vi "Serve Control Endpoint.vi"(5 "Response":refnum<class "Response.lvclass">, 7 "Request":refnum<class "Request.lvclass">, 8 "error in (no error)":errorcluster) -> (0 "error out":errorcluster, 2 "Handled?":bool)   [LabVIEW 2023, in "Server.lvclass"]
uses:
  Server.lvclass
  Request/Request.lvclass
  Response/Response.lvclass
  Response/Standard Response Messages.ctl
  e9d03b97-7d0a-453d-8c8e-3f8556095b4f.vi
  1685da64-af02-4367-9c77-a6898df52c71.vi
  d533b881-5725-4b61-bb0f-1b9536aa055f.vi
  68d5b38b-bcce-484c-a16b-74d95231e072.vi
  96f92e60-dc3c-449d-a1e9-fb4d73dbd9f4.vi
  e9d03b97-7d0a-453d-8c8e-3f8556095b4f.vi/bf0030c7-b76b-4182-9f9e-16cd2e366061.vi
  1685da64-af02-4367-9c77-a6898df52c71.vi/bf0030c7-b76b-4182-9f9e-16cd2e366061.vi
  d533b881-5725-4b61-bb0f-1b9536aa055f.vi/bf0030c7-b76b-4182-9f9e-16cd2e366061.vi
  68d5b38b-bcce-484c-a16b-74d95231e072.vi/bf0030c7-b76b-4182-9f9e-16cd2e366061.vi
  96f92e60-dc3c-449d-a1e9-fb4d73dbd9f4.vi/bf0030c7-b76b-4182-9f9e-16cd2e366061.vi
  Request/Get Request.vi
  Response/Set Body.vi
  Response/Set Content Type.vi
  Response/Set Status Code.vi
  Response/Send.vi
  Response/Private/Format Control Data Element.vi
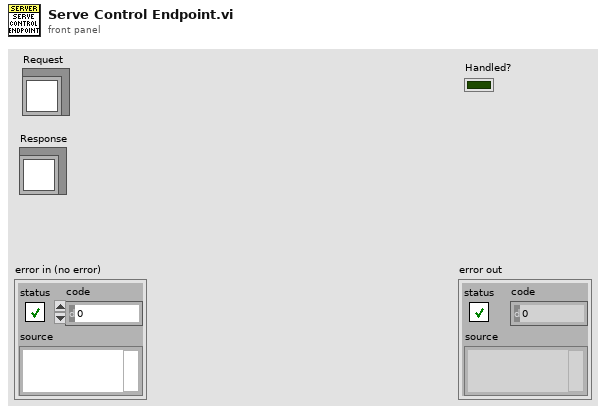
[diagram p1: front panel]
types:
  T1 = typedef "Server.lvclass/ObjectAttributes.ctl" = cluster{"Static Data":path, "MIME Types":variant, "Shutdown":bool, "API Queue":refnum<queue>, "ControlEndpoints":map{string, cluster{"Ref":refnum<vi>, "Mode":T2}}, "EventEndpoints":map{string, refnum<user-event>}}
  T2 = typedef "Server.lvclass/Control Ref Endpoint Access Mode.ctl" = enum16{"None", "Read/Write", "Read Only", "Write Only"}
  T3 = typedef "Request.ctl" = cluster{"Method":string, "URI":string, "Protocol":string, "Raw Path":string, "Query":string, "Fragment":string, "Raw Body":string, "Headers":variant, "Parameters":variant, "Body":variant, "Raw Header":string, "Path":string[]}
  T4 = map{string, cluster{"Ref":refnum<vi>, "Mode":T2}}
  T5 = typedef "Response.lvclass/Standard Response Messages.ctl" = u16
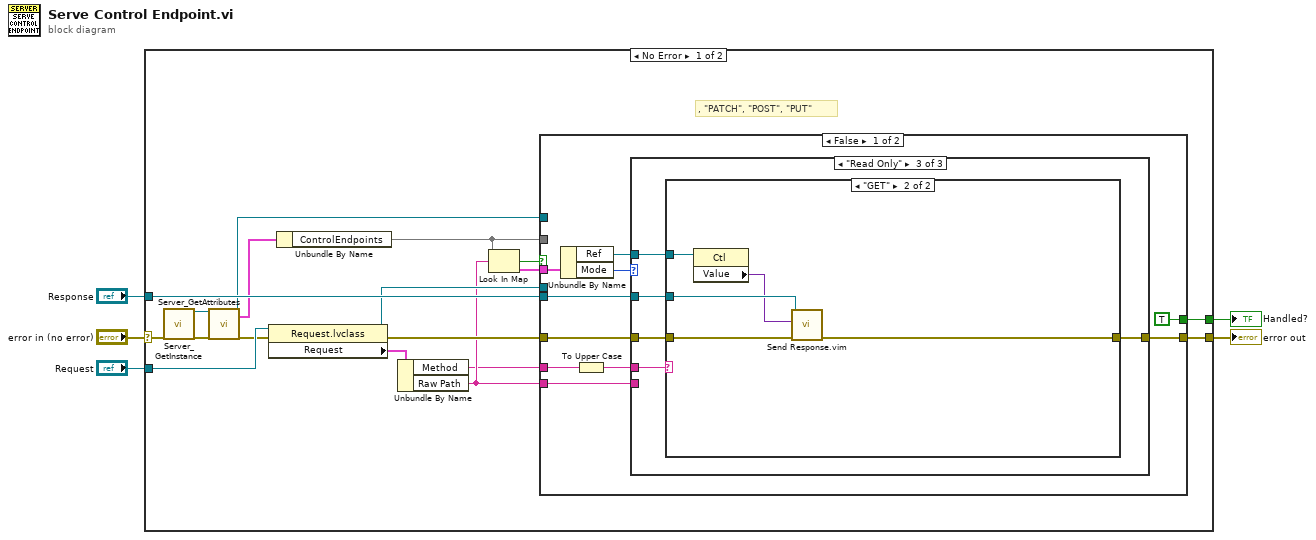
[diagram p0: block diagram]
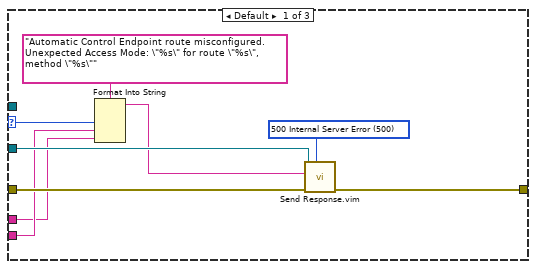
[diagram p2: hidden frame]
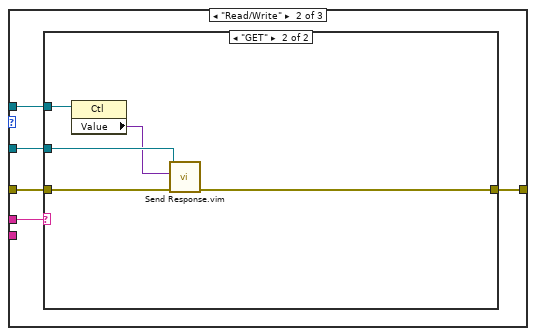
[diagram p3: hidden frame]
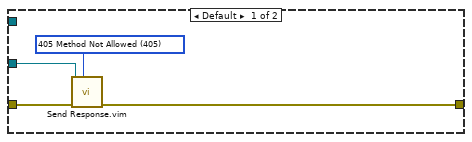
[diagram p4: hidden frame]
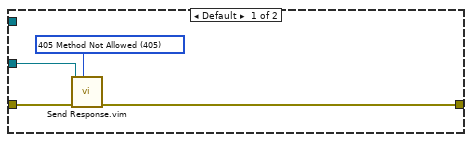
[diagram p5: hidden frame]
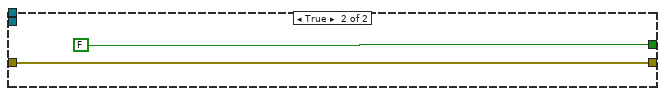
[diagram p6: hidden frame]
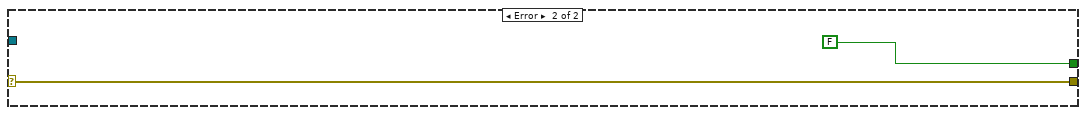
[diagram p7: hidden frame]
diagram:
  n1 = case shown="No Error" "error in (no error)" {
    selector: "error in (no error)" -> [w19 w74]
    tunnel: [w7 w74] -> w4
    tunnel: "Request" -> [w23 _]
    tunnel: "Response" -> [w20 _]
    tunnel: [w6 FALSE] -> w1
    frame No Error {
      # ", \"PATCH\", \"POST\", \"PUT\""
      n2 = call "Server_GetInstance.vi"("error in (no error)"=w19) -> ("reference out"=w15:refnum<class "Server.lvclass">, "error out"=w16:errorcluster)  [unwired: 14 in, 3 out]
      n3 = call "Server_GetAttributes.vi"("reference in"=w15, "error in (no error)"=w16) -> ("reference out"=w14:refnum<class "Server.lvclass">, "Data"=w17:T1, "error out"=w18:errorcluster)  [unwired: 14 in, 1 out]
      n4 = property class="Request.lvclass"(reference=w23, error in=w18) -> (reference out=w13:refnum<class "Request.lvclass">, error out=w21:errorcluster, "Request"=w22:T3)
      n5 = Unbundle By Name(w17) -> ("ControlEndpoints"=w12:T4)
      n6 = Unbundle By Name(w22) -> ("Method"=w8:string, "Raw Path"=w11:string)
      n7 = Look In Map(map=w12, key=w11) -> (key not found?=w10:bool, value=w9:cluster{"Ref":refnum<vi>, "Mode":T2})  [unwired: 1 in]
      n8 = case shown="False" w10 {
        tunnel: w21 -> [w32 w72]
        tunnel: w20 -> [w27 _]
        tunnel: w11 -> [w25 _]
        tunnel: w12 -> [_ _]
        tunnel: w14 -> [_ _]
        tunnel: w13 -> [_ _]
        tunnel: w9 -> [w33 _]
        tunnel: w8 -> [w30 _]
        tunnel: [w28 w72] -> w7
        tunnel: [TRUE FALSE] -> w6
        frame False {
          n9 = Unbundle By Name(w33) -> ("Ref"=w24:refnum<vi>, "Mode"=w31:T2)
          n10 = To Upper Case(1:w30) -> (0:w29:string)
          n11 = case shown="\"Read Only\"" w31 {
            selector: w31 -> [w38 _ _]
            tunnel: w32 -> [w42 w46 w60]
            tunnel: w29 -> [w35 w47 w61]
            tunnel: [w41 w45 w59] -> w28
            tunnel: w27 -> [w40 w44 w58]
            tunnel: w25 -> [w36 _ _]
            tunnel: w24 -> [_ w43 w57]
            frame Default {
              w39 = T5 500 items=["200 OK"=200, "201 Created"=201, "202 Accepted"=202, "203 Non-Authoritative Information"=203, "204 No Content"=204, "205 Reset Content"=205, "206 Partial Content"=206, "207 Multi-Status (WebDAV)"=207, "208 Already Reported (WebDAV)"=208, "226 IM Used (HTTP Delta encoding)"=226, "300 Multiple Choices"=300, "301 Moved Permanently"=301, "302 Found"=302, "303 See Other"=303, "304 Not Modified"=304, "305 Use Proxy Deprecated"=305, "307 Temporary Redirect"=307, "308 Permanent Redirect"=308, "400 Bad Request"=400, "401 Unauthorized"=401, "402 Payment Required"=402, "403 Forbidden"=403, "404 Not Found"=404, "405 Method Not Allowed"=405, "406 Not Acceptable"=406, "407 Proxy Authentication Required"=407, "408 Request Timeout"=408, "409 Conflict"=409, "410 Gone"=410, "411 Length Required"=411, "412 Precondition Failed"=412, "413 Content Too Large"=413, "414 URI Too Long"=414, "415 Unsupported Media Type"=415, "416 Range Not Satisfiable"=416, "417 Expectation Failed"=417, "418 I'm a teapot"=418, "421 Misdirected Request"=421, "422 Unprocessable Content (WebDAV)"=422, "423 Locked (WebDAV)"=423, "424 Failed Dependency (WebDAV)"=424, "425 Too Early Experimental"=425, "426 Upgrade Required"=426, "428 Precondition Required"=428, "429 Too Many Requests"=429, "431 Request Header Fields Too Large"=431, "451 Unavailable For Legal Reasons"=451, "500 Internal Server Error"=500, "501 Not Implemented"=501, "502 Bad Gateway"=502, "503 Service Unavailable"=503, "504 Gateway Timeout"=504, "505 HTTP Version Not Supported"=505, "506 Variant Also Negotiates"=506, "507 Insufficient Storage (WebDAV)"=507, "508 Loop Detected (WebDAV)"=508, "510 Not Extended"=510, "511 Network Authentication Required"=511] ("Status Code (200=OK)")
              n12 = Format Into String(format string="Automatic Control Endpoint route misconfigured. Unexpected Access Mode: \"%s\" for route \"%s\", method \"%s\"", w38, w36, w35) -> (resulting string=w37:string)  [unwired: 2 in, 1 out]
              n13 = call "Send Response.vim"("Status Code (200=OK)"=w39, "Error In"=w42, "Body (\"\")"=w37, "Response"=w40) -> ("Error Out"=w41:errorcluster)  [unwired: 7 in]
            }
            frame "Read/Write" {
              n14 = case shown="\"GET\"" w47 {
                tunnel: w46 -> [w51 w56]
                tunnel: [w50 w53] -> w45
                tunnel: w44 -> [w49 w54]
                tunnel: w43 -> [_ w55]
                frame Default {
                  w48 = T5 405 items=["200 OK"=200, "201 Created"=201, "202 Accepted"=202, "203 Non-Authoritative Information"=203, "204 No Content"=204, "205 Reset Content"=205, "206 Partial Content"=206, "207 Multi-Status (WebDAV)"=207, "208 Already Reported (WebDAV)"=208, "226 IM Used (HTTP Delta encoding)"=226, "300 Multiple Choices"=300, "301 Moved Permanently"=301, "302 Found"=302, "303 See Other"=303, "304 Not Modified"=304, "305 Use Proxy Deprecated"=305, "307 Temporary Redirect"=307, "308 Permanent Redirect"=308, "400 Bad Request"=400, "401 Unauthorized"=401, "402 Payment Required"=402, "403 Forbidden"=403, "404 Not Found"=404, "405 Method Not Allowed"=405, "406 Not Acceptable"=406, "407 Proxy Authentication Required"=407, "408 Request Timeout"=408, "409 Conflict"=409, "410 Gone"=410, "411 Length Required"=411, "412 Precondition Failed"=412, "413 Content Too Large"=413, "414 URI Too Long"=414, "415 Unsupported Media Type"=415, "416 Range Not Satisfiable"=416, "417 Expectation Failed"=417, "418 I'm a teapot"=418, "421 Misdirected Request"=421, "422 Unprocessable Content (WebDAV)"=422, "423 Locked (WebDAV)"=423, "424 Failed Dependency (WebDAV)"=424, "425 Too Early Experimental"=425, "426 Upgrade Required"=426, "428 Precondition Required"=428, "429 Too Many Requests"=429, "431 Request Header Fields Too Large"=431, "451 Unavailable For Legal Reasons"=451, "500 Internal Server Error"=500, "501 Not Implemented"=501, "502 Bad Gateway"=502, "503 Service Unavailable"=503, "504 Gateway Timeout"=504, "505 HTTP Version Not Supported"=505, "506 Variant Also Negotiates"=506, "507 Insufficient Storage (WebDAV)"=507, "508 Loop Detected (WebDAV)"=508, "510 Not Extended"=510, "511 Network Authentication Required"=511] ("Status Code (200=OK)")
                  n15 = call "Send Response.vim"("Status Code (200=OK)"=w48, "Error In"=w51, "Response"=w49) -> ("Error Out"=w50:errorcluster)  [unwired: 8 in]
                }
                frame "GET" {
                  n16 = property class="Ctl"(reference=w55) -> ("Value"=w52:variant)  [unwired: 1 in, 2 out]
                  n17 = call "Send Response.vim"("Error In"=w56, "Body (\"\")"=w52, "Response"=w54) -> ("Error Out"=w53:errorcluster)  [unwired: 8 in]
                }
              }
            }
            frame "Read Only" {
              n18 = case shown="\"GET\"" w61 {
                tunnel: w60 -> [w65 w70]
                tunnel: [w64 w67] -> w59
                tunnel: w58 -> [w63 w68]
                tunnel: w57 -> [_ w69]
                frame Default {
                  w62 = T5 405 items=["200 OK"=200, "201 Created"=201, "202 Accepted"=202, "203 Non-Authoritative Information"=203, "204 No Content"=204, "205 Reset Content"=205, "206 Partial Content"=206, "207 Multi-Status (WebDAV)"=207, "208 Already Reported (WebDAV)"=208, "226 IM Used (HTTP Delta encoding)"=226, "300 Multiple Choices"=300, "301 Moved Permanently"=301, "302 Found"=302, "303 See Other"=303, "304 Not Modified"=304, "305 Use Proxy Deprecated"=305, "307 Temporary Redirect"=307, "308 Permanent Redirect"=308, "400 Bad Request"=400, "401 Unauthorized"=401, "402 Payment Required"=402, "403 Forbidden"=403, "404 Not Found"=404, "405 Method Not Allowed"=405, "406 Not Acceptable"=406, "407 Proxy Authentication Required"=407, "408 Request Timeout"=408, "409 Conflict"=409, "410 Gone"=410, "411 Length Required"=411, "412 Precondition Failed"=412, "413 Content Too Large"=413, "414 URI Too Long"=414, "415 Unsupported Media Type"=415, "416 Range Not Satisfiable"=416, "417 Expectation Failed"=417, "418 I'm a teapot"=418, "421 Misdirected Request"=421, "422 Unprocessable Content (WebDAV)"=422, "423 Locked (WebDAV)"=423, "424 Failed Dependency (WebDAV)"=424, "425 Too Early Experimental"=425, "426 Upgrade Required"=426, "428 Precondition Required"=428, "429 Too Many Requests"=429, "431 Request Header Fields Too Large"=431, "451 Unavailable For Legal Reasons"=451, "500 Internal Server Error"=500, "501 Not Implemented"=501, "502 Bad Gateway"=502, "503 Service Unavailable"=503, "504 Gateway Timeout"=504, "505 HTTP Version Not Supported"=505, "506 Variant Also Negotiates"=506, "507 Insufficient Storage (WebDAV)"=507, "508 Loop Detected (WebDAV)"=508, "510 Not Extended"=510, "511 Network Authentication Required"=511] ("Status Code (200=OK)")
                  n19 = call "Send Response.vim"("Status Code (200=OK)"=w62, "Error In"=w65, "Response"=w63) -> ("Error Out"=w64:errorcluster)  [unwired: 8 in]
                }
                frame "GET" {
                  n20 = property class="Ctl"(reference=w69) -> ("Value"=w66:variant)  [unwired: 1 in, 2 out]
                  n21 = call "Send Response.vim"("Error In"=w70, "Body (\"\")"=w66, "Response"=w68) -> ("Error Out"=w67:errorcluster)  [unwired: 8 in]
                }
              }
            }
          }
        }
        frame True {
        }
      }
    }
    frame Error {
    }
  }
  "error out" <- w4
  "Handled?" <- w1
